vi "NumberToSign.vi"(8 "error in (no error)":errorcluster, 10 "Number":i32) -> (0 "error out":errorcluster, 2 "Display":string)   [LabVIEW 2015, in "Panel_UI.lvclass"]
uses:
  Panel_UI.lvclass
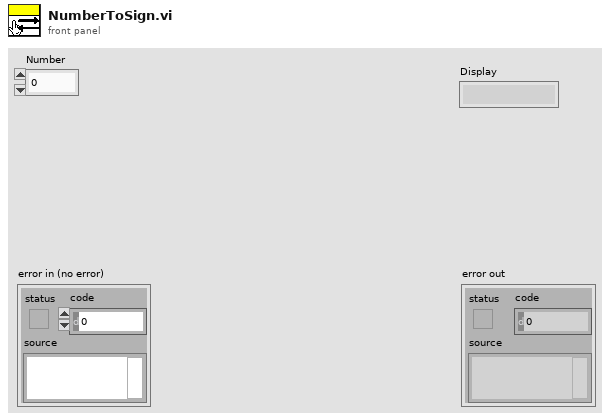
[diagram p1: front panel]
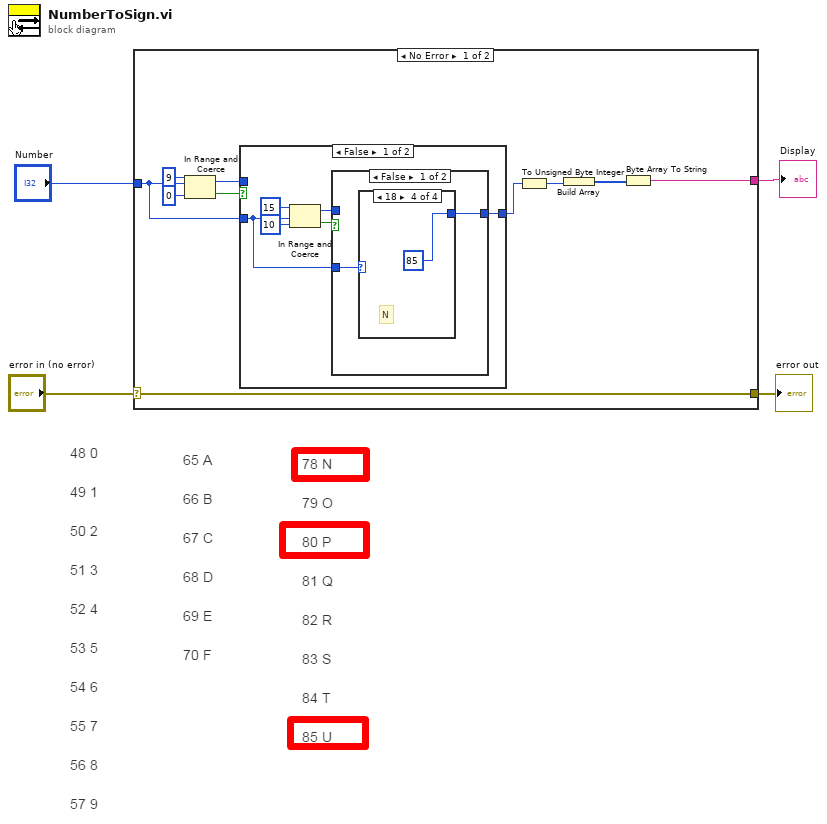
[diagram p0: block diagram]
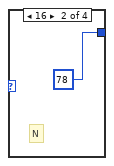
[diagram p3: hidden frame]
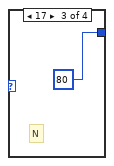
[diagram p4: hidden frame]
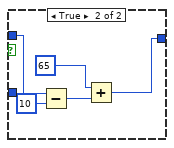
[diagram p5: hidden frame]
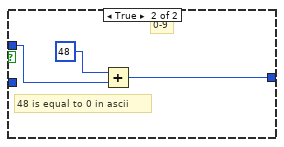
[diagram p6: hidden frame]
diagram:
  n1 = case shown="No Error" "error in (no error)" {
    selector: "error in (no error)" -> [w14 w34]
    tunnel: [w14 w34] -> w3
    tunnel: "Number" -> [w8 _]
    tunnel: [w7 _] -> w1
    frame No Error {
      n2 = In Range and Coerce(upper limit=9, x=w8, lower limit=0) -> (coerced(x)=w9:i32, In Range?=w10:bool)
      n3 = case shown="False" w10 {
        tunnel: w9 -> [_ w32]
        tunnel: [w15 w31] -> w6
        tunnel: w8 -> [w16 _]
        frame False {
          n4 = In Range and Coerce(upper limit=15, x=w16, lower limit=10) -> (coerced(x)=w17:i32, In Range?=w18:bool)
          n5 = case shown="False" w18 {
            tunnel: w17 -> [_ w30]
            tunnel: [w21 w26] -> w15
            tunnel: w16 -> [w22 _]
            frame False {
              n6 = case shown="18" w22 {
                tunnel: [_ 78 80 85] -> w21
                frame Default {
                }
                frame 16 {
                  # "N"
                }
                frame 17 {
                  # "N"
                }
                frame 18 {
                  # "N"
                }
              }
            }
            frame True {
              n7 = Subtract(x=w30, y=10) -> (x-y=w27:i32)
              n8 = Add(x=65, y=w27) -> (x+y=w26:i32)
            }
          }
        }
        frame True {
          # "0-9"
          # "48 is equal to 0 in ascii"
          n9 = Add(x=48, y=w32) -> (x+y=w31:i32)
        }
      }
      n10 = To Unsigned Byte Integer(number=w6) -> (unsigned 8bit integer=w5:u8)
      n11 = Build Array(w5) -> (w13:u8[])
      n12 = Byte Array To String(unsigned byte array=w13) -> (string=w7:string)
    }
    frame Error {
    }
  }
  "error out" <- w3
  "Display" <- w1
